vi "Electronic Procedure Debug.vi"() -> ()   [LabVIEW 2017]
panel:
  in  "stop":bool
  in  "CTAH outlet temperature":dbl
  in  "mass flow rate":dbl
  in  "CTAH frequency":dbl
  in  "desired power":dbl
  in  "pump frequency":dbl
  # "Do NOT run this during an experiment!"
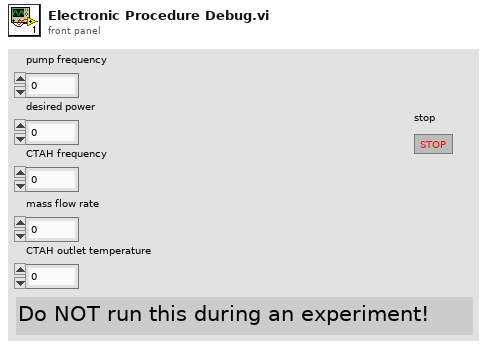
[diagram p1: front panel]
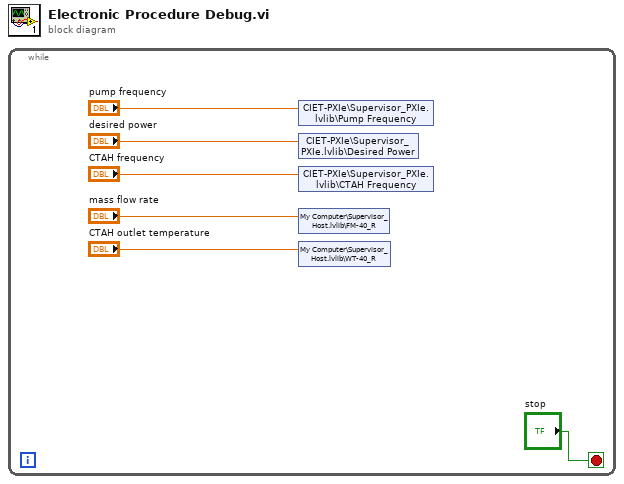
[diagram p0: block diagram]
diagram:
  n1 = while {
    stop <- "stop" stop-if-true
    n2 = shared-variable "CIET-PXIe\\Supervisor_PXIe.lvlib\\Pump Frequency"("pump frequency") -> ()  [unwired: 1 in, 1 out]
    n3 = shared-variable "CIET-PXIe\\Supervisor_PXIe.lvlib\\Desired Power"("desired power") -> ()  [unwired: 1 in, 1 out]
    n4 = shared-variable "CIET-PXIe\\Supervisor_PXIe.lvlib\\CTAH Frequency"("CTAH frequency") -> ()  [unwired: 1 in, 1 out]
    n5 = shared-variable "My Computer\\Supervisor_Host.lvlib\\FM-40_R"("mass flow rate") -> ()  [unwired: 1 in, 1 out]
    n6 = shared-variable "My Computer\\Supervisor_Host.lvlib\\WT-40_R"("CTAH outlet temperature") -> ()  [unwired: 1 in, 1 out]
  }
